vi "PH_Beckhoff.publish digital DIM service.vi"(5 "error in":errorcluster, 6 "Value":bool, 7 "Quality ok?":bool, 8 "Service ID":i32) -> (0 "error out":errorcluster)   [LabVIEW 2014, in "PH_Beckhoff.lvlib"]
doc: "This VI is used to publish a boolean DIM service including quality."
uses:
  PH_Beckhoff.lvlib
  CSlibraries-extern/DimLVEvent/LVDimInterface/LVDimInterface.lvlib
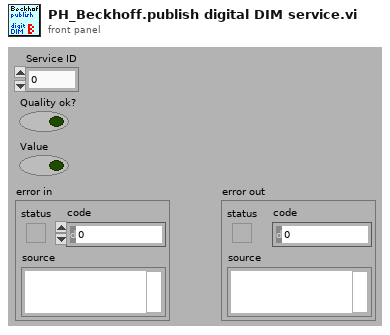
[diagram p1: front panel]
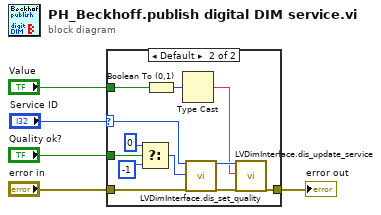
[diagram p0: block diagram]
diagram:
  n1 = case shown="Default" "Service ID" {
    selector: "Service ID" -> [_ w7]
    tunnel: "Quality ok?" -> [_ w15]
    tunnel: "Value" -> [_ w11]
    tunnel: "error in" -> [w6 w9]
    tunnel: [w6 w8] -> w4
    frame -1 {
    }
    frame Default {
      n2 = Select(t=0, s=w15, f=-1) -> (s? t:f=w14:i32)
      n3 = Boolean To (0,1)(Boolean=w11) -> (0, 1=w10:i16)
      n4 = Type Cast(x=w10) -> (*(type *) &x=w16:string)  [unwired: 1 in]
      n5 = call "LVDimInterface.dis_set_quality.vi"("my_serviceID"=w7, "quality"=w14, "error in (no error)"=w9) -> ("my_serviceID (out)"=w17:i32, "error out"=w18:errorcluster)  [unwired: 15 in]
      n6 = call "LVDimInterface.dis_update_service.vi"("my_serviceID"=w17, "data"=w16, "error in (no error)"=w18) -> ("error out"=w8:errorcluster)  [unwired: 14 in, 2 out]
    }
  }
  "error out" <- w4
